vi "GetOffsetFormulasINI.vi"(0 "configuration file path":path, 1 "error in (no error)":errorcluster) -> (2 "file path":path, 3 "HorzOffsetFormula":string, 4 "VertOffsetFormula":string, 5 "error out":errorcluster)   [LabVIEW 2012]
uses:
  <vilib>/Utility/config.llb/Read Key (String).vi
  <vilib>/Utility/config.llb/NI_LVConfig.lvlib
panel:
  # "Input value must be \"Distance\""
  # "Output must be \"HorzOffset\" or \"VertOffset\" respectively."
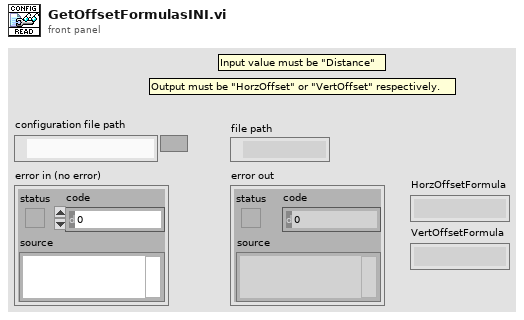
[diagram p1: front panel]
types:
  T1 = typedef "NI_LVConfig.lvlib/Config Data RefNum.ctl" = refnum<k1>
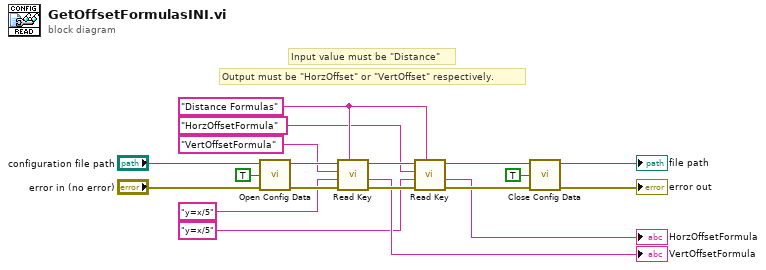
[diagram p0: block diagram]
diagram:
  w11 = "Distance Formulas"
  # "Output must be \"HorzOffset\" or \"VertOffset\" respectively."
  # "Input value must be \"Distance\""
  n1 = call <vilib>:"Open Config Data.vi"("error in (no error)"="error in (no error)", "create file if necessary (T)"=TRUE, "configuration file path"="configuration file path") -> ("error out"=w16:errorcluster, "refnum"=w17:T1)  [unwired: 6 in, 1 out]
  n2 = call-poly <vilib>:"Read Key.vi"("section"=w11, "error in (no error)"=w16, "default value"="y=x/5", "key"="VertOffsetFormula", "refnum"=w17) -> ("error out"=w14:errorcluster, "value"=→"VertOffsetFormula":string, "refnum out"=w15:T1)  [unwired: 3 in, 1 out]
  n3 = call-poly <vilib>:"Read Key.vi"("section"=w11, "error in (no error)"=w14, "default value"="y=x/5", "key"="HorzOffsetFormula", "refnum"=w15) -> ("error out"=w13:errorcluster, "value"=→"HorzOffsetFormula":string, "refnum out"=w12:T1)  [unwired: 3 in, 1 out]
  n4 = call <vilib>:"Close Config Data.vi"("error in (no error)"=w13, "write file if changed (T)"=TRUE, "refnum"=w12) -> ("error out"=→"error out":errorcluster, "file path"=→"file path":path)  [unwired: 7 in]
